vi "PRL C37 Data Reader Wrapper.vi"(10 "Initialize Time":bool, 11 "Pseudo PDC ID":i32) -> (0 "Digital Data":bool[](array[boolean]), 1 "Analog Data":sgl[](array[numeric]), 2 "Phasor Data":csg[](array[numeric]), 3 "Time Stamp":timestamp, 4 "Relative System Clock (ms)":dbl, 5 "PMU Status":T1(array[cluster]), 6 "dt (ms)":dbl, 7 "Data OK":bool)   [LabVIEW 2018, in "S3DK.lvlib" / "PMU Recorder Light.lvlib"]
uses:
  PMU Recorder Light.lvlib
  Statnett C37.118 DLL/Statnett C37.118 DLL.lvclass
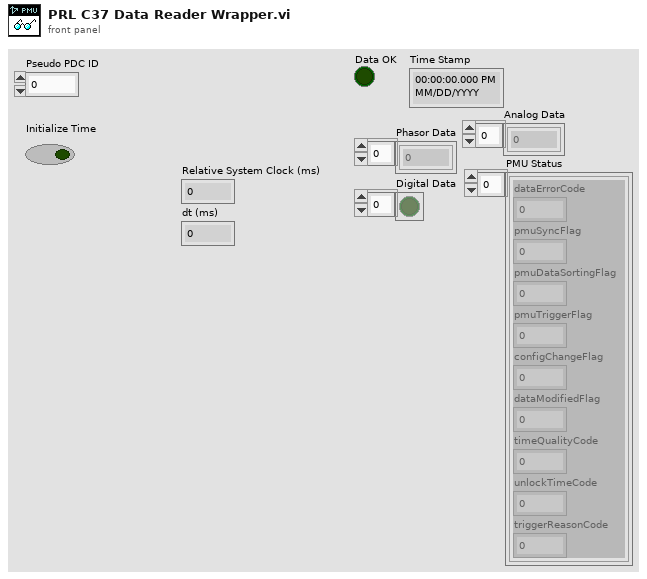
[diagram p1: front panel]
types:
  T1 = cluster{"dataErrorCode":u8, "pmuSyncFlag":u8, "pmuDataSortingFlag":u8, "pmuTriggerFlag":u8, "configChangeFlag":u8, "dataModifiedFlag":u8, "timeQualityCode":u8, "unlockTimeCode":u8, "triggerReasonCode":u8}[]
  T2 = cluster{"Frequency":sgl, "Frequency Delta":sgl, "Phasor Data":csg[], "Analog Data":sgl[], "Digital Data":bool[]}[]
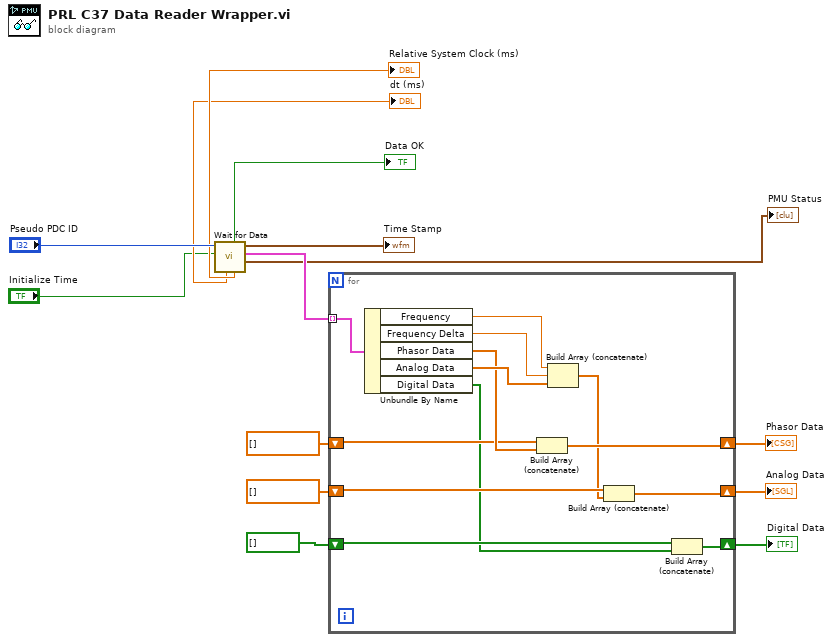
[diagram p0: block diagram]
diagram:
  n1 = call "Wait for Data.vi"("Initialize Time"="Initialize Time", "Pseudo PDC ID"="Pseudo PDC ID") -> ("PMU Status"=→"PMU Status":T1, "PMU Data"=w11:T2, "Time Stamp"=→"Time Stamp":timestamp, "Relative System Clock (ms)"=→"Relative System Clock (ms)":dbl, "Data OK"=→"Data OK":bool, "dt (ms)"=→"dt (ms)":dbl)  [unwired: 3 in, 1 out]
  n2 = for {
    tunnel: w11 -> [w27] mode=indexing
    shift-right: [w21] -> w7
    shift-left: csg[] [] -> [w22]
    shift-right: [w20] -> w6
    shift-left: sgl[] [] -> [w19]
    shift-right: [w17] -> w5
    shift-left: bool[] [] -> [w18]
    n3 = Unbundle By Name(w27) -> ("Frequency"=w26:sgl, "Frequency Delta"=w25:sgl, "Phasor Data"=w23:csg[], "Analog Data"=w24:sgl[], "Digital Data"=w15:bool[])
    n4 = Build Array (concatenate)(w22, w23) -> (w21:csg[])
    n5 = Build Array (concatenate)(w26, w25, w24) -> (w16:sgl[])
    n6 = Build Array (concatenate)(w19, w16) -> (w20:sgl[])
    n7 = Build Array (concatenate)(w18, w15) -> (w17:bool[])
  }
  "Phasor Data" <- w7
  "Analog Data" <- w6
  "Digital Data" <- w5
